vi "Global_firing.vi"() -> ()   [LabVIEW 2013]
panel:
  in  "Firing":bool
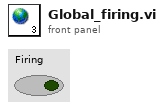
[diagram p1: front panel]
diagram:
